vi "user32_IsMenu.vi"(0 "hMenu":u32, 11 "错误输入（无错误）":errorcluster) -> (4 "dup hMenu":u32, 6 "IsMenu?":bool, 15 "错误输出":errorcluster)   [LabVIEW 2011]
doc: "该函数确定一个句柄是否为菜单句柄。"
uses:
  user32.dll
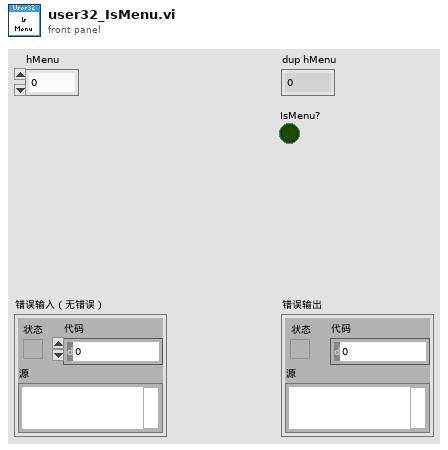
[diagram p1: front panel]
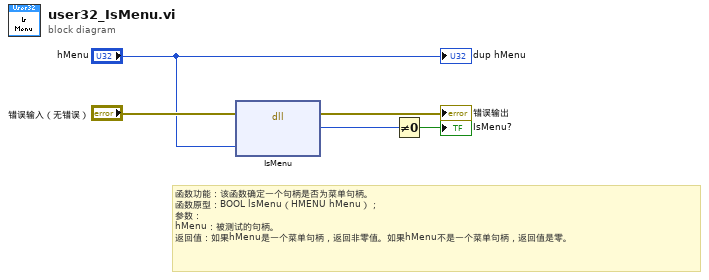
[diagram p0: block diagram]
diagram:
  # "函数功能：该函数确定一个句柄是否为菜单句柄。\n函数原型：BOOL lsMenu（HMENU hMenu）；\n参数：\nhMenu：被测试的句柄。\n返回值：如果hMenu是一个菜单句柄，返回非零值。如果hMenu不是一个菜单句柄，返回值是零。"
  n1 = dll-call lib="user32.dll" fn="IsMenu"(error in="错误输入（无错误）", "hMenu"="hMenu") -> (error out=→"错误输出":errorcluster, "Bool"=w2:u8)  [unwired: 3 in, 1 out]
  n2 = Not Equal To 0?(x=w2) -> (x != 0?=→"IsMenu?":bool)
  "dup hMenu" <- "hMenu"
